vi "Exponential.vi"   [LabVIEW 2018, in "NI_Matrix.lvlib"]
doc: "Computes the exponential of the input matrix."
uses:
  NI_Matrix.lvlib
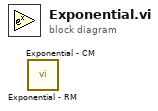
[diagram p0: block diagram]
diagram:
  n1 = call "Exponential - RM.vi"() -> ()  [unwired: 1 in, 1 out]
  n2 = call "Exponential - CM.vi"() -> ()  [unwired: 1 in, 1 out]
